vi "WriteWaveformTriggered.vi"(7 "trigger edge":i32(ring)=10280 items=["Rising"=10280, "Falling"=10171], 8 "error in (no error)":errorcluster, 9 "Trigger source":tag="/Dev3/PFI0", 10 "waveform in":waveform(dbl), 11 "physical channel":tag="Dev2/ao3") -> (0 "error out":errorcluster, 3 "task out":refnum<k21>)   [LabVIEW 2018]
uses:
  <vilib>/DAQmx/write.llb/DAQmx Write (Analog Wfm 1Chan NSamp).vi
  <vilib>/DAQmx/create/channels.llb/DAQmx Create Channel (AO-Voltage-Basic).vi
  <vilib>/DAQmx/configure/timing.llb/DAQmx Timing (Sample Clock).vi
  <vilib>/DAQmx/configure/trigger.llb/DAQmx Start Trigger (Digital Edge).vi
  <vilib>/DAQmx/miscellaneous.llb/DAQmx Fill In Error Info.vi
panel:
  in  "stop":bool
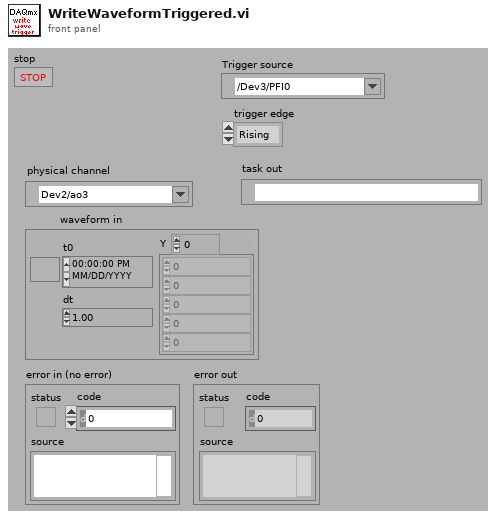
[diagram p1: front panel]
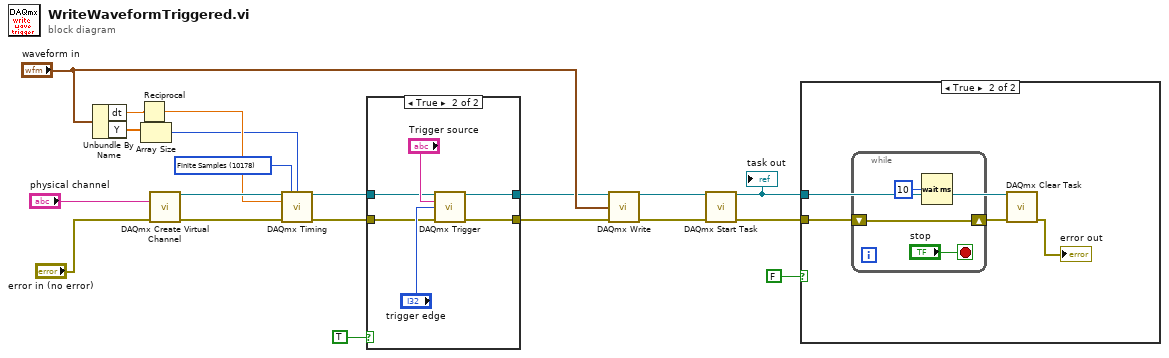
[diagram p0: block diagram]
diagram:
  w9 = 10178 items=["Finite Samples"=10178, "Continuous Samples"=10123, "Hardware Timed Single Point"=12522] ("sample mode")
  n1 = Unbundle By Name("waveform in") -> ("dt"=w12:dbl, "Y"=w13:dbl[])
  n2 = Reciprocal(x=w12) -> (1/x=w11:dbl)
  n3 = Array Size(array=w13) -> (size(s)=w10:i32)
  n4 = call-poly <vilib>:"DAQmx Create Virtual Channel.vi"("physical channels"="physical channel", "error in"="error in (no error)") -> ("task out"=w19:refnum<k21>, "error out"=w17:errorcluster)  [unwired: 12 in]
  n5 = call-poly <vilib>:"DAQmx Timing.vi"("task/channels in"=w19, "sample mode"=w9, "samples per channel"=w10, "rate"=w11, "error in"=w17) -> ("task out"=w7:refnum<k21>, "error out"=w2:errorcluster)  [unwired: 9 in]
  n6 = case shown="True" TRUE {
    tunnel: w7 -> [w22 w26]
    tunnel: [w22 w25] -> w6
    tunnel: [w21 w24] -> w3
    tunnel: w2 -> [w21 w23]
    frame False {
    }
    frame True {
      n7 = call-poly <vilib>:"DAQmx Trigger.vi"("task/channels in"=w26, "source"="Trigger source", "edge"="trigger edge", "error in"=w23) -> ("task out"=w25:refnum<k21>, "error out"=w24:errorcluster)  [unwired: 10 in]
    }
  }
  n8 = call-poly <vilib>:"DAQmx Write.vi"("task/channels in"=w6, "data"="waveform in", "error in"=w3) -> ("task out"=w5:refnum<k21>, "error out"=w4:errorcluster)  [unwired: 10 in, 1 out]
  n9 = call <vilib>:"DAQmx Start Task.vi"("task/channels in"=w5, "error in"=w4) -> ("task out"=w15:refnum<k21>, "error out"=w16:errorcluster)  [unwired: 12 in]
  "task out" <- w15
  n10 = case shown="True" FALSE {
    tunnel: w16 -> [_ w30]
    tunnel: w15 -> [_ w31]
    frame False {
    }
    frame True {
      n11 = while {
        shift-right: [w33] -> w29
        shift-left: w30 -> [w33]
        stop <- "stop" stop-if-true
        n12 = Wait (ms)(milliseconds to wait=u32 10) -> ()  [unwired: 1 out]
      }
      n13 = call <vilib>:"DAQmx Clear Task.vi"("task in"=w31, "error in"=w29) -> ("error out"=→"error out":errorcluster)  [unwired: 13 in]
    }
  }
